vi "Resource Path.vi"(8 "error in (no error)":errorcluster, 10 "resource file name":string, 11 "data dir":path) -> (0 "error out":errorcluster, 3 "path":path)   [LabVIEW 2014, in "lvprj2html.lvlib"]
uses:
  lvprj2html.lvlib
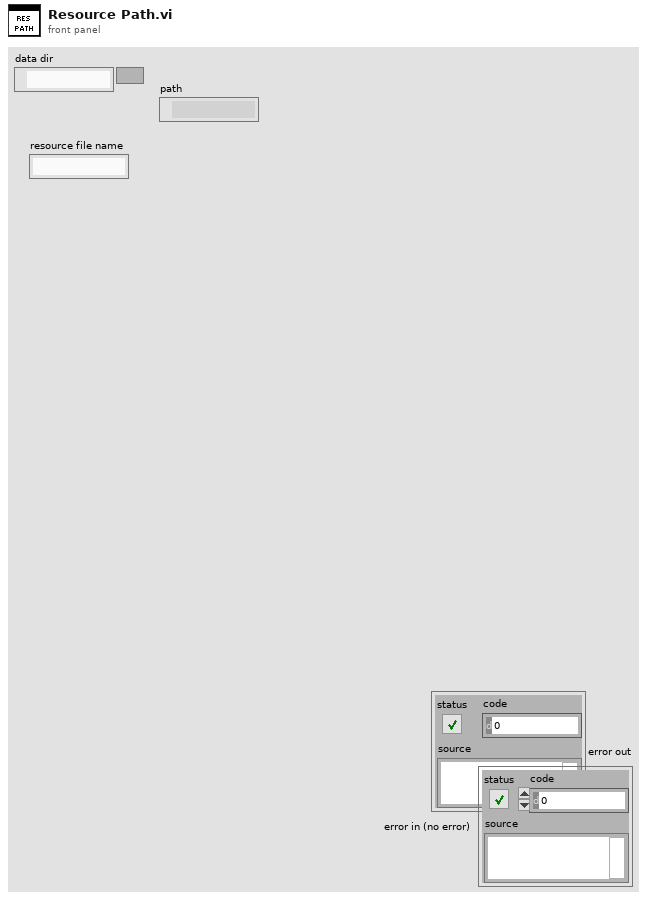
[diagram p1: front panel]
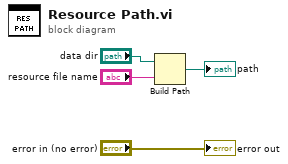
[diagram p0: block diagram]
diagram:
  n1 = Build Path(base path="data dir", name or relative path="resource file name") -> (appended path=→"path":path)
  "error out" <- "error in (no error)"
